vi "_UI.vi"(10 "WindowType":T1(tab), 11 "UI_ProgressDlg.lvclass":refnum<class "UI_ProgressDlg.lvclass">) -> ()   [LabVIEW 2014, in "UI_ProgressDlg.lvlib" / "UI_ProgressDlg.lvclass"]
doc: "UI_ProgressDlg.lvclass"
uses:
  UI_ProgressDlg.lvclass
  <vilib>/Utility/miscctls.llb/LVRangeTypeDef.ctl
  UI_ProgressDlg.lvclass/UI_ProgressDlg.ctl
panel:
  out "Inforamtion":string
  out "Prograss":dbl(slide) scale=0.0..100.0
  out "Time Elapsed(BuzyWnd)":string
  out "Time Elapsed":string
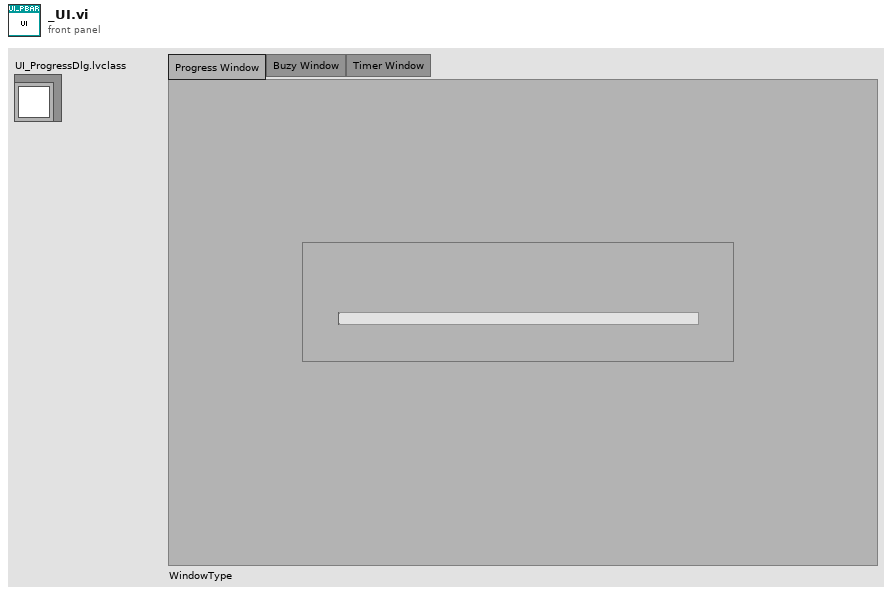
[diagram p1: front panel]
types:
  T1 = enum32{"Progress Window", "Buzy Window", "Timer Window"}
  T2 = typedef "LVRangeTypeDef.ctl" = cluster{"Minimum":dbl, "Maximum":dbl, "Increment":dbl, "Minor Increment":dbl, "Start":dbl}
  T3 = cluster{"Information":string, "Scale.Range":T2, "progress":dbl, "StartTime":timestamp}
  T4 = typedef "UI_ProgressDlg.lvlib/UI_ProgressDlg.lvclass/DEF-Data.ctl" = cluster{"stopped?":bool}
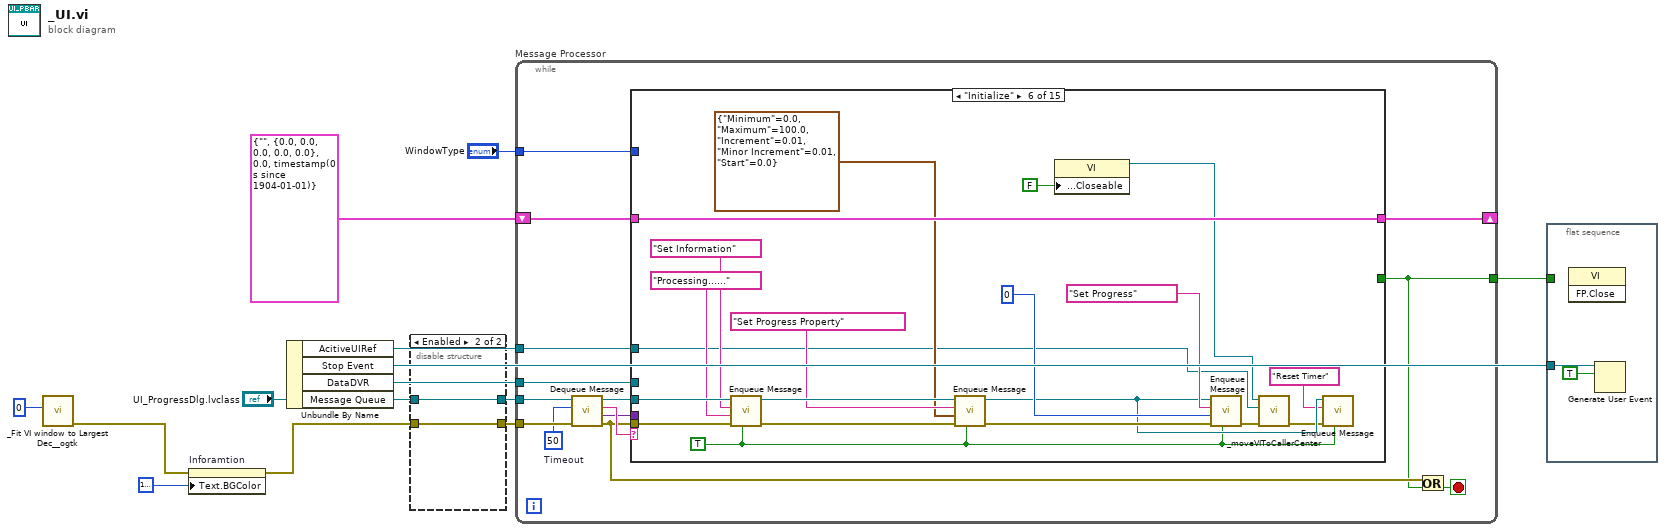
[diagram p0: block diagram]
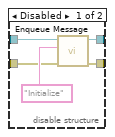
[diagram p2: hidden frame]
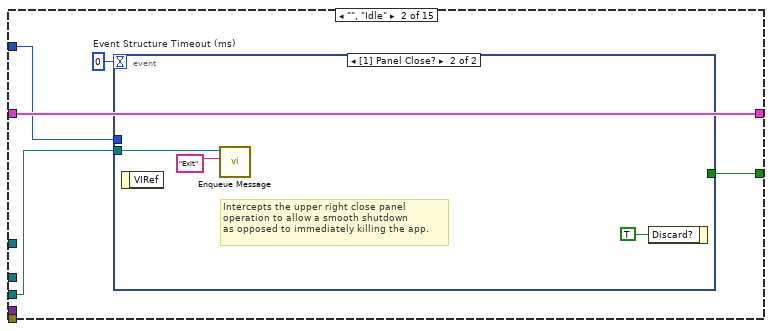
[diagram p4: hidden frame]
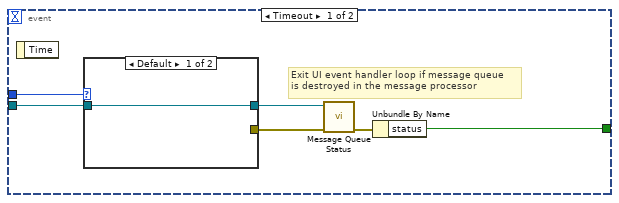
[diagram p5: hidden frame]
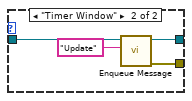
[diagram p6: hidden frame]
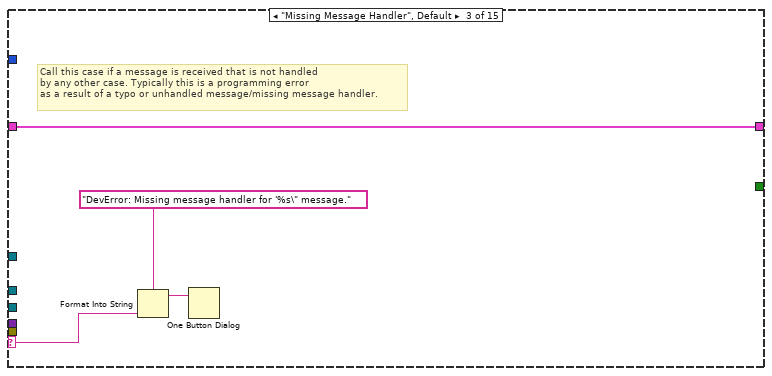
[diagram p7: hidden frame]
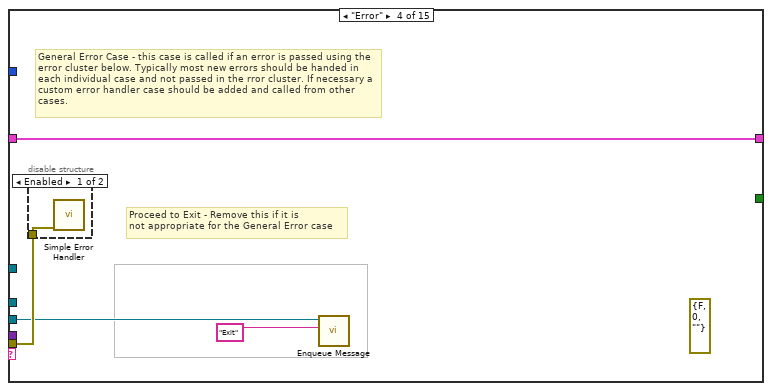
[diagram p8: hidden frame]
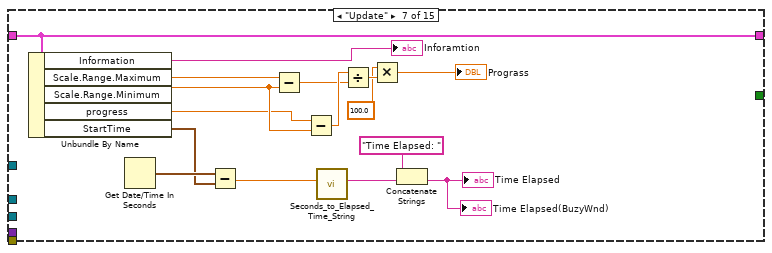
[diagram p11: hidden frame]
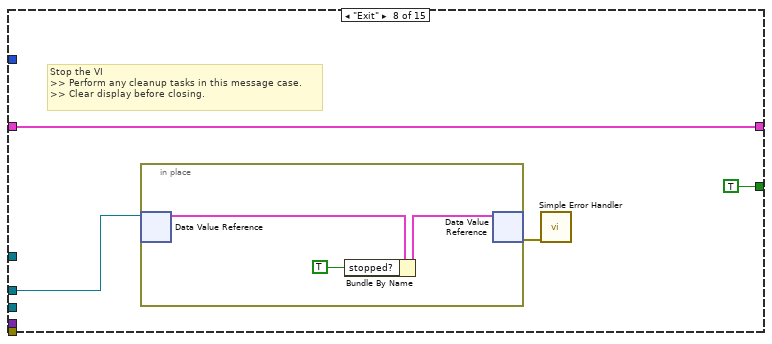
[diagram p12: hidden frame]
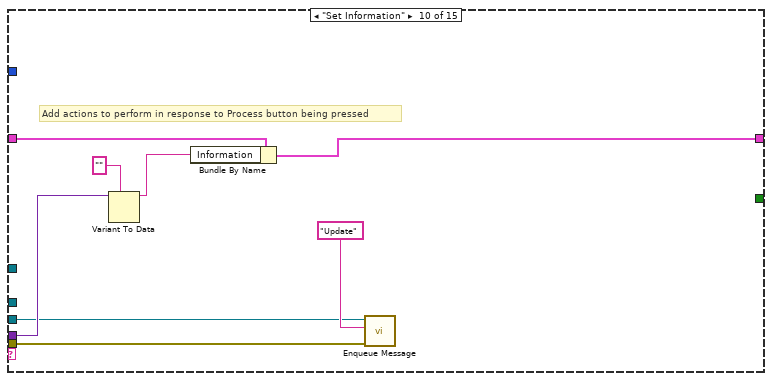
[diagram p14: hidden frame]
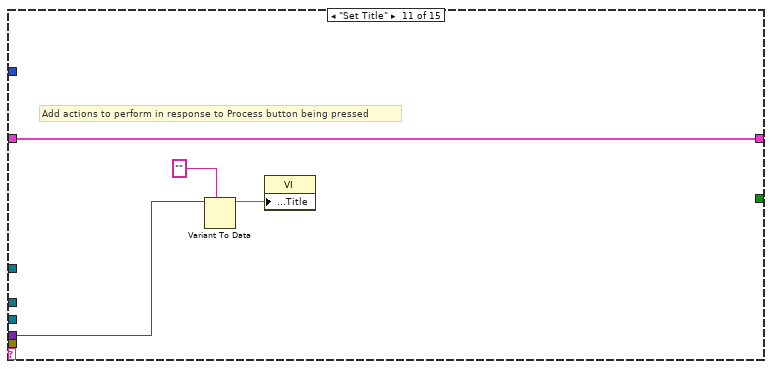
[diagram p15: hidden frame]
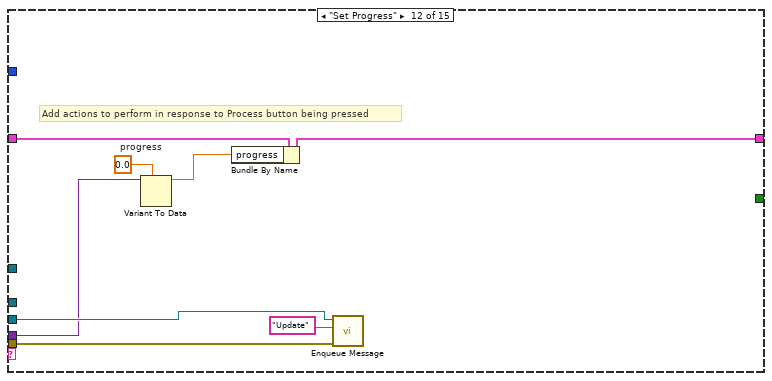
[diagram p16: hidden frame]
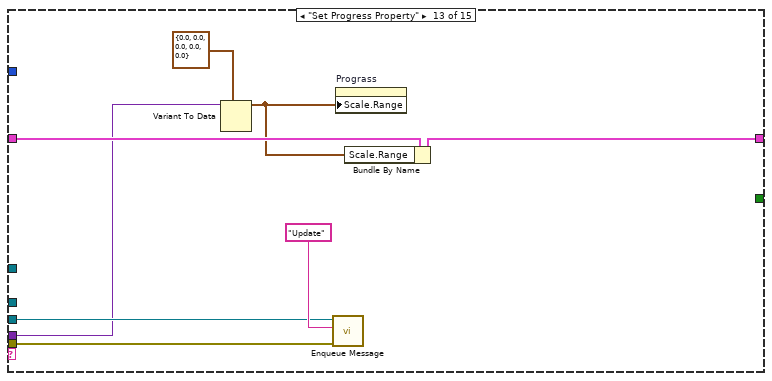
[diagram p17: hidden frame]
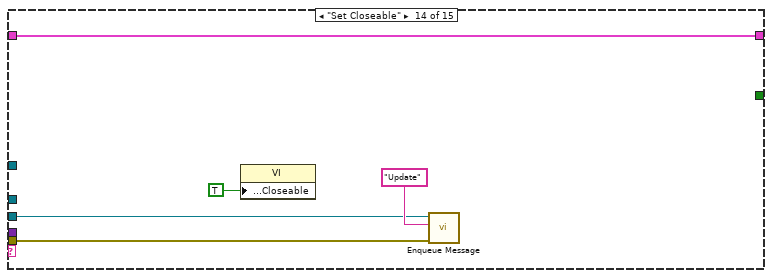
[diagram p18: hidden frame]
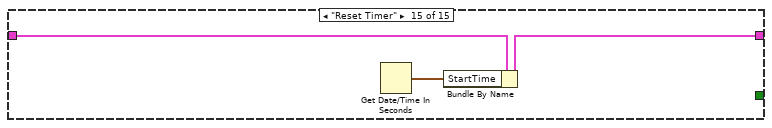
[diagram p19: hidden frame]
diagram:
  n1 = call "_Fit VI window to Largest Dec__ogtk.vi"("border spacing (2 px)"=0) -> ("error out"=w5:errorcluster)  [unwired: 5 in, 1 out]
  n2 = property on="Inforamtion" class="Str"(error in=w5, "Text.BGColor"=u32 16777216) -> (error out=w4:errorcluster)  [unwired: 1 in, 1 out]
  n3 = Unbundle By Name("UI_ProgressDlg.lvclass") -> ("AcitiveUIRef"=w1:refnum<vi>, "Stop Event"=w2:refnum<user-event>, "DataDVR"=w3:refnum<data-value>, "Message Queue"=w10:refnum<queue>)
  n4 = disable-structure shown="Enabled" {
    disable-tunnel: [w18 w21] -> w13
    disable-tunnel: [w17 w20] -> w12
    disable-tunnel: w10 -> [w16 w21]
    disable-tunnel: w4 -> [w15 w20]
    frame Disabled {
      n5 = call "Enqueue Message.vi"("error in (no error)"=w15, "Message"="Initialize", "Message Queue"=w16) -> ("error out"=w17:errorcluster, "dup Message Queue"=w18:refnum<queue>)  [unwired: 7 in]
    }
    frame Enabled {
    }
  }
  n6 = while "Message Processor" {
    tunnel: w13 -> [w32]
    shift-left: T3 {"Information"="", "Scale.Range"={"Minimum"=0.0, "Maximum"=0.0, "Increment"=0.0, "Minor Increment"=0.0, "Start"=0.0}, "progress"=0.0, "StartTime"=timestamp(0 s since 1904-01-01)} ("state variables") -> [w35]
    shift-right: [w34] -> _
    tunnel: w12 -> [w31]
    tunnel: [w25] -> w9
    tunnel: "WindowType" -> [w24]
    tunnel: w3 -> [w23]
    tunnel: w1 -> [w22]
    stop <- w27 stop-if-true
    w28 = 50  # Timeout
    n7 = call "Dequeue Message.vi"("error in (no error)"=w31, "timeout in ms (-1)"=w28, "Message Queue"=w32) -> ("error out"=w26:errorcluster, "Message Data"=w29:variant, "Message"=w30:string, "dup Message Queue"=w33:refnum<queue>)  [unwired: 4 in, 1 out]
    n8 = case shown="\"Initialize\"" w30 {
      selector: w30 -> [_ _ w58 _ _ _ _ _ _ _ _ _ _ _ _]
      tunnel: [w36 w41 w59 w63 w65 w85 w101 w105 w109 w116 w121 w127 w135 w142 w144] -> w34
      tunnel: w35 -> [w36 w41 w59 w63 w65 w85 w101 w105 w109 w117 w121 w129 w137 w142 w145]
      tunnel: w33 -> [_ w39 _ w60 _ w83 _ _ _ w112 _ w124 w132 w139 _]
      tunnel: w26 -> [_ _ _ w61 _ w84 _ _ _ w113 _ w126 w133 w140 _]
      tunnel: w29 -> [_ _ _ _ _ _ _ _ _ w115 w120 w123 w131 _ _]
      tunnel: [_ w37 _ _ _ _ _ TRUE ("Discard?") _ _ _ _ _ _ _] -> w25
      tunnel: w24 -> [_ w38 _ _ _ _ _ _ _ _ _ _ _ _ _]
      tunnel: w23 -> [_ _ _ _ _ _ _ w103 _ _ _ _ _ _ _]
      tunnel: w22 -> [_ _ _ _ _ w70 _ _ _ _ _ _ _ _ _]
      frame "---------- Framework Operations ----------" {
        # "Dummy case to add a seperator in the Case Structure menu"
      }
      frame "", "Idle" {
        w40 = 0  # Event Structure Timeout (ms)
        n9 = event shown="[1] Panel Close?" {
          selector: _ -> [_ _]
          dyn-events: _ -> [_ _]
          timeout: w40 -> [_ _]
          tunnel: w39 -> [w44 w53]
          tunnel: w38 -> [w46 _]
          tunnel: [w42 _] -> w37
          event Timeout {
            # "Exit UI event handler loop if message queue\nis destroyed in the message processor"
            n10 = event-data() -> ()  [unwired: 2 out]
            n11 = case shown="Default" w46 {
              tunnel: [w48 w52] -> w45
              tunnel: w44 -> [w48 w51]
              tunnel: [_ w49] -> w43
              frame Default {
              }
              frame "Timer Window" {
                n12 = call "Enqueue Message.vi"("Message"="Update", "Message Queue"=w51) -> ("error out"=w49:errorcluster, "dup Message Queue"=w52:refnum<queue>)  [unwired: 8 in]
              }
            }
            n13 = call "Message Queue Status.vi"("error in (no error)"=w43, "Message Queue"=w45) -> ("error out"=w47:errorcluster)  [unwired: 8 in, 1 out]
            n14 = Unbundle By Name(w47) -> ("status"=w42:bool)
          }
          event Panel Close? {
            # "Intercepts the upper right close panel\noperation to allow a smooth shutdown\nas opposed to immediately killing the app."
            n15 = event-data() -> ()  [unwired: 2 out]
            n16 = call "Enqueue Message.vi"("Message"="Exit", "Message Queue"=w53) -> ()  [unwired: 8 in, 2 out]
            n17 = event-data("Discard?"=TRUE) -> ()  [unwired: 1 in, 1 out]
          }
        }
      }
      frame "Missing Message Handler", Default {
        # "Call this case if a message is received that is not handled \nby any other case. Typically this is a programming error\nas a result of a typo or unhandled message/missing message handler."
        n18 = Format Into String(format string="DevError: Missing message handler for '%s\" message." ("message"), w58) -> (resulting string=w56:string)  [unwired: 2 in, 1 out]
        n19 = One Button Dialog(message=w56) -> ()  [unwired: 2 out]
      }
      frame "Error" {
        (unwired) errorcluster {"status"=FALSE, "code"=0, "source"=""} ("error out")
        # "Proceed to Exit - Remove this if it is\nnot appropriate for the General Error case"
        # "General Error Case - this case is called if an error is passed using the error cluster below. Typically most new errors should be handed in each individual case and not passed in the rror cluster. If necessary a custom error handler case should be added and called from other cases."
        n20 = disable-structure shown="Enabled" {
          disable-tunnel: w61 -> [w64 _]
          frame Enabled {
            n21 = call <vilib>:"Simple Error Handler.vi"("error in (no error)"=w64) -> ()  [unwired: 1 in, 8 out]
          }
          frame Disabled {
          }
        }
        n22 = call "Enqueue Message.vi"("Message"="Exit", "Message Queue"=w60) -> ()  [unwired: 8 in, 2 out]
      }
      frame "---------- Generic Operations ----------" {
        # "Dummy case to add a seperator in the Case Structure menu"
      }
      frame "Initialize" {
        w66 = TRUE ("Priority Message? (F)")
        n23 = call "Enqueue Message.vi"("Priority Message? (F)"=w66, "error in (no error)"=w84, "Message Data"="Processing......" ("Inforamtion"), "Message"="Set Information" ("Inforamtion"), "Message Queue"=w83) -> ("error out"=w82:errorcluster, "dup Message Queue"=w81:refnum<queue>)  [unwired: 5 in]
        n24 = call "Enqueue Message.vi"("Priority Message? (F)"=w66, "error in (no error)"=w82, "Message Data"=T2 {"Minimum"=0.0, "Maximum"=100.0, "Increment"=0.01, "Minor Increment"=0.01, "Start"=0.0} ("Scale.Range"), "Message"="Set Progress Property" ("Inforamtion"), "Message Queue"=w81) -> ("error out"=w80:errorcluster, "dup Message Queue"=w69:refnum<queue>)  [unwired: 5 in]
        n25 = property class="VI"("Front Panel.Closeable"=FALSE ("Front Panel Window:Closeable")) -> (reference out=w71:refnum<vi>)  [unwired: 2 in, 1 out]
        n26 = call "Enqueue Message.vi"("Priority Message? (F)"=w66, "error in (no error)"=w80, "Message Data"=u32 0 ("Prograss"), "Message"="Set Progress" ("Inforamtion"), "Message Queue"=w69) -> ("error out"=w72:errorcluster)  [unwired: 5 in, 1 out]
        n27 = call "_moveVIToCallerCenter.vi"("error in (no error)"=w72, "CallerVI in"=w70, "VI in"=w71) -> ("error out"=w68:errorcluster)  [unwired: 6 in, 2 out]
        n28 = call "Enqueue Message.vi"("Priority Message? (F)"=w66, "error in (no error)"=w68, "Message"="Reset Timer", "Message Queue"=w69) -> ()  [unwired: 6 in, 2 out]
      }
      frame "Update" {
        n29 = Unbundle By Name(w101) -> ("Information"=→"Inforamtion":string, "Scale.Range.Maximum"=w100:dbl, "Scale.Range.Minimum"=w99:dbl, "progress"=w94:dbl, "StartTime"=w90:timestamp)
        n30 = Get Date/Time In Seconds() -> (seconds since 1Jan1904=w91:timestamp)
        n31 = Subtract(x=w91, y=w90) -> (x-y=w89:dbl)
        n32 = Subtract(x=w100, y=w99) -> (x-y=w97:dbl)
        n33 = Subtract(x=w94, y=w99) -> (x-y=w98:dbl)
        n34 = call "Seconds_to_Elapsed_Time_String.vi"("# Seconds (0)"=w89) -> ("Elapsed Time (00:00:00)"=w88:string)  [unwired: 10 in]
        n35 = Divide(x=w98, y=w97) -> (x/y=w96:dbl)
        n36 = Multiply(x=100.0, y=w96) -> (x*y=→"Prograss":dbl)
        n37 = Concatenate Strings("Time Elapsed: " ("string"), w88) -> (→"Time Elapsed" →"Time Elapsed(BuzyWnd)":string)
      }
      frame "Exit" {
        # "Stop the VI\n>> Perform any cleanup tasks in this message case.\n>> Clear display before closing."
        n38 = in-place {
          n39 = in-place-dvr #1(w103) -> (w108:T4)  [unwired: 1 out]
          n40 = Bundle By Name(cluster=w108, "stopped?"=TRUE) -> (w107:T4)
          n41 = in-place-dvr #1(w107) -> (w102:errorcluster)  [unwired: 1 out]
        }
        n42 = call <vilib>:"Simple Error Handler.vi"("error in (no error)"=w102) -> ()  [unwired: 4 in, 5 out]
      }
      frame "---------- Application Operations ----------" {
      }
      frame "Set Information" {
        # "Add actions to perform in response to Process button being pressed"
        n43 = Variant To Data(type="", Variant=w115) -> (data=w110:string)  [unwired: 1 in, 1 out]
        n44 = Bundle By Name(cluster=w117, "Information"=w110) -> (w116:T3)
        n45 = call "Enqueue Message.vi"("error in (no error)"=w113, "Message"="Update" ("message name"), "Message Queue"=w112) -> ()  [unwired: 7 in, 2 out]
      }
      frame "Set Title" {
        # "Add actions to perform in response to Process button being pressed"
        n46 = Variant To Data(type="", Variant=w120) -> (data=w119:string)  [unwired: 1 in, 1 out]
        n47 = property class="VI"("Front Panel.Title"=w119) -> ()  [unwired: 2 in, 2 out]
      }
      frame "Set Progress" {
        w128 = 0.0  # progress
        # "Add actions to perform in response to Process button being pressed"
        n48 = Variant To Data(type=w128, Variant=w123) -> (data=w122:dbl)  [unwired: 1 in, 1 out]
        n49 = Bundle By Name(cluster=w129, "progress"=w122) -> (w127:T3)
        n50 = call "Enqueue Message.vi"("error in (no error)"=w126, "Message"="Update" ("message name"), "Message Queue"=w124) -> ()  [unwired: 7 in, 2 out]
      }
      frame "Set Progress Property" {
        n51 = Variant To Data(type=T2 {"Minimum"=0.0, "Maximum"=0.0, "Increment"=0.0, "Minor Increment"=0.0, "Start"=0.0} ("Scale.Range"), Variant=w131) -> (data=w130:T2)  [unwired: 1 in, 1 out]
        n52 = call "Enqueue Message.vi"("error in (no error)"=w133, "Message"="Update" ("message name"), "Message Queue"=w132) -> ()  [unwired: 7 in, 2 out]
        n53 = property on="Prograss" class="Slide (strict)"("Scale.Range"=w130) -> ()  [unwired: 2 in, 2 out]
        n54 = Bundle By Name(cluster=w137, "Scale.Range"=w130) -> (w135:T3)
      }
      frame "Set Closeable" {
        n55 = property class="VI"("Front Panel.Closeable"=TRUE ("Front Panel Window:Closeable")) -> ()  [unwired: 2 in, 2 out]
        n56 = call "Enqueue Message.vi"("error in (no error)"=w140, "Message"="Update" ("message name"), "Message Queue"=w139) -> ()  [unwired: 7 in, 2 out]
      }
      frame "Reset Timer" {
        n57 = Get Date/Time In Seconds() -> (seconds since 1Jan1904=w143:timestamp)
        n58 = Bundle By Name(cluster=w145, "StartTime"=w143) -> (w144:T3)
      }
    }
    n59 = Or(x=w26, y=w25) -> (x .or. y?=w27:bool)
  }
  n60 = flat-sequence {
    tunnel: w9 -> [_]
    tunnel: w2 -> [w147]
    frame #0 {
      n61 = invoke class="VI" method="FP.Close"() -> ()  [unwired: 3 in, 3 out]
      n62 = Generate User Event(user event=w147, event data cluster=TRUE ("event data")) -> ()  [unwired: 2 in, 2 out]
    }
  }
